vi "example_02_convert.vi"() -> ()   [LabVIEW 2015, in "lv-unit-conversion.lvlib"] (continued)
"b"=2684519.537696173, "c"=1.0, "d"=0.0, "underlying_def"="", "description"=""}, {"symbol"="hp[metric].h", "name"="metric-horsepower hour", "dimension"="L2M/T2", "is_si_unit"=TRUE, "category"="derived", "base_unit"="J", "conversion_reference"="DERIVED", "is_exact"=TRUE, "a"=0.0, "b"=2647795.5, "c"=1.0, "d"=0.0, "underlying_def"="", "description"=""}, {"symbol"="kW.h", "name"="kilowatt hour", "dimension"="L2M/T2", "is_si_unit"=TRUE, "category"="derived", "base_unit"="J", "conversion_reference"="DERIVED", "is_exact"=TRUE, "a"=0.0, "b"=3600000.0, "c"=1.0, "d"=0.0, "underlying_def"="", "description"=""}, {"symbol"="MW.h", "name"="megawatt hour", "dimension"="L2M/T2", "is_si_unit"=TRUE, "category"="derived", "base_unit"="J", "conversion_reference"="DERIVED", "is_exact"=TRUE, "a"=0.0, "b"=3600000000.0, "c"=1.0, "d"=0.0, "underlying_def"="", "description"=""}, {"symbol"="TW.h", "name"="terrawatt hour", "dimension"="L2M/T2", "is_si_unit"=TRUE, "category"="derived", "base_unit"="J", "conversion_reference"="DERIVED", "is_exact"=TRUE, "a"=0.0, "b"=3600000000000000.0, "c"=1.0, "d"=0.0, "underlying_def"="", "description"=""}, {"symbol"="1000 lbf.ft", "name"="thousand foot pound-force", "dimension"="L2M/T2", "is_si_unit"=TRUE, "category"="derived", "base_unit"="N.m", "conversion_reference"="DERIVED", "is_exact"=TRUE, "a"=0.0, "b"=1355.8179483314004, "c"=1.0, "d"=0.0, "underlying_def"="", "description"=""}, {"symbol"="daN.m", "name"="dekanewton metre", "dimension"="L2M/T2", "is_si_unit"=TRUE, "category"="derived", "base_unit"="N.m", "conversion_reference"="DERIVED", "is_exact"=TRUE, "a"=0.0, "b"=10.0, "c"=1.0, "d"=0.0, "underlying_def"="", "description"=""}, {"symbol"="dN.m", "name"="decinewton metre", "dimension"="L2M/T2", "is_si_unit"=TRUE, "category"="derived", "base_unit"="N.m", "conversion_reference"="DERIVED", "is_exact"=TRUE, "a"=0.0, "b"=0.1, "c"=1.0, "d"=0.0, "underlying_def"="", "description"=""}, {"symbol"="kgf.m", "name"="thousand gram-force metre", "dimension"="L2M/T2", "is_si_unit"=TRUE, "category"="derived", "base_unit"="N.m", "conversion_reference"="DERIVED", "is_exact"=TRUE, "a"=0.0, "b"=9.80665, "c"=1.0, "d"=0.0, "underlying_def"="", "description"=""}, {"symbol"="kN.m", "name"="kilonewton metre", "dimension"="L2M/T2", "is_si_unit"=TRUE, "category"="derived", "base_unit"="N.m", "conversion_reference"="DERIVED", "is_exact"=TRUE, "a"=0.0, "b"=1000.0, "c"=1.0, "d"=0.0, "underlying_def"="", "description"=""}, {"symbol"="lbf.ft", "name"="foot pound-force", "dimension"="L2M/T2", "is_si_unit"=TRUE, "category"="derived", "base_unit"="N.m", "conversion_reference"="DERIVED", "is_exact"=TRUE, "a"=0.0, "b"=1.3558179483314003, "c"=1.0, "d"=0.0, "underlying_def"="", "description"=""}, {"symbol"="lbf.in", "name"="inch pound-force", "dimension"="L2M/T2", "is_si_unit"=TRUE, "category"="derived", "base_unit"="N.m", "conversion_reference"="DERIVED", "is_exact"=TRUE, "a"=0.0, "b"=0.1129848290276167, "c"=1.0, "d"=0.0, "underlying_def"="", "description"=""}, {"symbol"="lbm.ft2/s2", "name"="pound-mass square foot per second squared", "dimension"="L2M/T2", "is_si_unit"=TRUE, "category"="derived", "base_unit"="N.m", "conversion_reference"="DERIVED", "is_exact"=TRUE, "a"=0.0, "b"=0.0421401100938048, "c"=1.0, "d"=0.0, "underlying_def"="", "description"=""}, {"symbol"="pdl.ft", "name"="foot poundal", "dimension"="L2M/T2", "is_si_unit"=TRUE, "category"="derived", "base_unit"="N.m", "conversion_reference"="DERIVED", "is_exact"=TRUE, "a"=0.0, "b"=0.0421401100938048, "c"=1.0, "d"=0.0, "underlying_def"="", "description"=""}, {"symbol"="tonf[US].ft", "name"="US ton-force foot", "dimension"="L2M/T2", "is_si_unit"=TRUE, "category"="derived", "base_unit"="N.m", "conversion_reference"="DERIVED", "is_exact"=TRUE, "a"=0.0, "b"=2711.635896662801, "c"=1.0, "d"=0.0, "underlying_def"="", "description"=""}, {"symbol"="tonf[US].mi", "name"="US ton-force mile", "dimension"="L2M/T2", "is_si_unit"=TRUE, "category"="derived", "base_unit"="N.m", "conversion_reference"="DERIVED", "is_exact"=TRUE, "a"=0.0, "b"=14317437.534379588, "c"=1.0, "d"=0.0, "underlying_def"="", "description"=""}, {"symbol"="aJ", "name"="attojoule", "dimension"="L2M/T2", "is_si_unit"=TRUE, "category"="prefixed", "base_unit"="J", "conversion_reference"="DERIVED", "is_exact"=TRUE, "a"=0.0, "b"=1e-18, "c"=1.0, "d"=0.0, "underlying_def"="", "description"=""}, {"symbol"="ccal[th]", "name"="hundredth of calorie", "dimension"="L2M/T2", "is_si_unit"=TRUE, "category"="prefixed", "base_unit"="J", "conversion_reference"="DERIVED", "is_exact"=TRUE, "a"=0.0, "b"=0.04184, "c"=1.0, "d"=0.0, "underlying_def"="", "description"=""}, {"symbol"="ceV", "name"="centielectronvolt", "dimension"="L2M/T2", "is_si_unit"=TRUE, "category"="prefixed", "base_unit"="J", "conversion_reference"="DERIVED", "is_exact"=TRUE, "a"=0.0, "b"=1.602176487e-21, "c"=1.0, "d"=0.0, "underlying_def"="", "description"=""}, {"symbol"="cJ", "name"="centijoule", "dimension"="L2M/T2", "is_si_unit"=TRUE, "category"="prefixed", "base_unit"="J", "conversion_reference"="DERIVED", "is_exact"=TRUE, "a"=0.0, "b"=0.01, "c"=1.0, "d"=0.0, "underlying_def"="", "description"=""}, {"symbol"="dcal[th]", "name"="tenth of calorie", "dimension"="L2M/T2", "is_si_unit"=TRUE, "category"="prefixed", "base_unit"="J", "conversion_reference"="DERIVED", "is_exact"=TRUE, "a"=0.0, "b"=0.4184, "c"=1.0, "d"=0.0, "underlying_def"="", "description"=""}, {"symbol"="deV", "name"="decielectronvolt", "dimension"="L2M/T2", "is_si_unit"=TRUE, "category"="prefixed", "base_unit"="J", "conversion_reference"="DERIVED", "is_exact"=TRUE, "a"=0.0, "b"=1.602176487e-20, "c"=1.0, "d"=0.0, "underlying_def"="", "description"=""}, {"symbol"="dJ", "name"="decijoule", "dimension"="L2M/T2", "is_si_unit"=TRUE, "category"="prefixed", "base_unit"="J", "conversion_reference"="DERIVED", "is_exact"=TRUE, "a"=0.0, "b"=0.1, "c"=1.0, "d"=0.0, "underlying_def"="", "description"=""}, {"symbol"="Ecal[th]", "name"="million million million calorie", "dimension"="L2M/T2", "is_si_unit"=TRUE, "category"="prefixed", "base_unit"="J", "conversion_reference"="DERIVED", "is_exact"=TRUE, "a"=0.0, "b"=4.184e+18, "c"=1.0, "d"=0.0, "underlying_def"="", "description"=""}, {"symbol"="EeV", "name"="exaelectronvolt", "dimension"="L2M/T2", "is_si_unit"=TRUE, "category"="prefixed", "base_unit"="J", "conversion_reference"="DERIVED", "is_exact"=TRUE, "a"=0.0, "b"=0.1602176487, "c"=1.0, "d"=0.0, "underlying_def"="", "description"=""}, {"symbol"="EJ", "name"="exajoule", "dimension"="L2M/T2", "is_si_unit"=TRUE, "category"="prefixed", "base_unit"="J", "conversion_reference"="DERIVED", "is_exact"=TRUE, "a"=0.0, "b"=1e+18, "c"=1.0, "d"=0.0, "underlying_def"="", "description"=""}, {"symbol"="fcal[th]", "name"="femtocalorie", "dimension"="L2M/T2", "is_si_unit"=TRUE, "category"="prefixed", "base_unit"="J", "conversion_reference"="DERIVED", "is_exact"=TRUE, "a"=0.0, "b"=4.184e-15, "c"=1.0, "d"=0.0, "underlying_def"="", "description"=""}, {"symbol"="feV", "name"="femtoelectronvolt", "dimension"="L2M/T2", "is_si_unit"=TRUE, "category"="prefixed", "base_unit"="J", "conversion_reference"="DERIVED", "is_exact"=TRUE, "a"=0.0, "b"=1.602176487e-34, "c"=1.0, "d"=0.0, "underlying_def"="", "description"=""}, {"symbol"="fJ", "name"="femtojoule", "dimension"="L2M/T2", "is_si_unit"=TRUE, "category"="prefixed", "base_unit"="J", "conversion_reference"="DERIVED", "is_exact"=TRUE, "a"=0.0, "b"=1e-15, "c"=1.0, "d"=0.0, "underlying_def"="", "description"=""}, {"symbol"="Gcal[th]", "name"="thousand million calorie", "dimension"="L2M/T2", "is_si_unit"=TRUE, "category"="prefixed", "base_unit"="J", "conversion_reference"="DERIVED", "is_exact"=TRUE, "a"=0.0, "b"=4184000000.0, "c"=1.0, "d"=0.0, "underlying_def"="", "description"=""}, {"symbol"="GeV", "name"="gigaelectronvolt", "dimension"="L2M/T2", "is_si_unit"=TRUE, "category"="prefixed", "base_unit"="J", "conversion_reference"="DERIVED", "is_exact"=TRUE, "a"=0.0, "b"=1.602176487e-10, "c"=1.0, "d"=0.0, "underlying_def"="", "description"=""}, {"symbol"="GJ", "name"="gigajoule", "dimension"="L2M/T2", "is_si_unit"=TRUE, "category"="prefixed", "base_unit"="J", "conversion_reference"="DERIVED", "is_exact"=TRUE, "a"=0.0, "b"=1000000000.0, "c"=1.0, "d"=0.0, "underlying_def"="", "description"=""}, {"symbol"="kcal[th]", "name"="thousand calorie", "dimension"="L2M/T2", "is_si_unit"=TRUE, "category"="prefixed", "base_unit"="J", "conversion_reference"="DERIVED", "is_exact"=TRUE, "a"=0.0, "b"=4184.0, "c"=1.0, "d"=0.0, "underlying_def"="", "description"="thermochemical calorie"}, {"symbol"="keV", "name"="kiloelectronvolt", "dimension"="L2M/T2", "is_si_unit"=TRUE, "category"="prefixed", "base_unit"="J", "conversion_reference"="DERIVED", "is_exact"=TRUE, "a"=0.0, "b"=1.602176487e-16, "c"=1.0, "d"=0.0, "underlying_def"="", "description"=""}, {"symbol"="kJ", "name"="kilojoule", "dimension"="L2M/T2", "is_si_unit"=TRUE, "category"="prefixed", "base_unit"="J", "conversion_reference"="DERIVED", "is_exact"=TRUE, "a"=0.0, "b"=1000.0, "c"=1.0, "d"=0.0, "underlying_def"="", "description"=""}, {"symbol"="mcal[th]", "name"="thousandth of calorie", "dimension"="L2M/T2", "is_si_unit"=TRUE, "category"="prefixed", "base_unit"="J", "conversion_reference"="DERIVED", "is_exact"=TRUE, "a"=0.0, "b"=0.004184, "c"=1.0, "d"=0.0, "underlying_def"="", "description"=""}, {"symbol"="Mcal[th]", "name"="million calorie", "dimension"="L2M/T2", "is_si_unit"=TRUE, "category"="prefixed", "base_unit"="J", "conversion_reference"="DERIVED", "is_exact"=TRUE, "a"=0.0, "b"=4184000.0, "c"=1.0, "d"=0.0, "underlying_def"="", "description"=""}, {"symbol"="MeV", "name"="megaelectronvolt", "dimension"="L2M/T2", "is_si_unit"=TRUE, "category"="prefixed", "base_unit"="J", "conversion_reference"="DERIVED", "is_exact"=TRUE, "a"=0.0, "b"=1.602176487e-13, "c"=1.0, "d"=0.0, "underlying_def"="", "description"=""}, {"symbol"="meV", "name"="millielectronvolt", "dimension"="L2M/T2", "is_si_unit"=TRUE, "category"="prefixed", "base_unit"="J", "conversion_reference"="DERIVED", "is_exact"=TRUE, "a"=0.0, "b"=1.602176487e-22, "c"=1.0, "d"=0.0, "underlying_def"="", "description"=""}, {"symbol"="mJ", "name"="millijoule", "dimension"="L2M/T2", "is_si_unit"=TRUE, "category"="prefixed", "base_unit"="J", "conversion_reference"="DERIVED", "is_exact"=TRUE, "a"=0.0, "b"=0.001, "c"=1.0, "d"=0.0, "underlying_def"="", "description"=""}, {"symbol"="MJ", "name"="megajoule", "dimension"="L2M/T2", "is_si_unit"=TRUE, "category"="prefixed", "base_unit"="J", "conversion_reference"="DERIVED", "is_exact"=TRUE, "a"=0.0, "b"=1000000.0, "c"=1.0, "d"=0.0, "underlying_def"="", "description"=""}, {"symbol"="ncal[th]", "name"="nanocalorie", "dimension"="L2M/T2", "is_si_unit"=TRUE, "category"="prefixed", "base_unit"="J", "conversion_reference"="DERIVED", "is_exact"=TRUE, "a"=0.0, "b"=4.184e-09, "c"=1.0, "d"=0.0, "underlying_def"="", "description"=""}, {"symbol"="neV", "name"="nanoelectronvolt", "dimension"="L2M/T2", "is_si_unit"=TRUE, "category"="prefixed", "base_unit"="J", "conversion_reference"="DERIVED", "is_exact"=TRUE, "a"=0.0, "b"=1.602176487e-28, "c"=1.0, "d"=0.0, "underlying_def"="", "description"=""}, {"symbol"="nJ", "name"="nanojoule", "dimension"="L2M/T2", "is_si_unit"=TRUE, "category"="prefixed", "base_unit"="J", "conversion_reference"="DERIVED", "is_exact"=TRUE, "a"=0.0, "b"=1e-09, "c"=1.0, "d"=0.0, "underlying_def"="", "description"=""}, {"symbol"="pcal[th]", "name"="picocalorie", "dimension"="L2M/T2", "is_si_unit"=TRUE, "category"="prefixed", "base_unit"="J", "conversion_reference"="DERIVED", "is_exact"=TRUE, "a"=0.0, "b"=4.184e-12, "c"=1.0, "d"=0.0, "underlying_def"="", "description"=""}, {"symbol"="peV", "name"="picoelectronvolt", "dimension"="L2M/T2", "is_si_unit"=TRUE, "category"="prefixed", "base_unit"="J", "conversion_reference"="DERIVED", "is_exact"=TRUE, "a"=0.0, "b"=1.602176487e-31, "c"=1.0, "d"=0.0, "underlying_def"="", "description"=""}, {"symbol"="pJ", "name"="picojoule", "dimension"="L2M/T2", "is_si_unit"=TRUE, "category"="prefixed", "base_unit"="J", "conversion_reference"="DERIVED", "is_exact"=TRUE, "a"=0.0, "b"=1e-12, "c"=1.0, "d"=0.0, "underlying_def"="", "description"=""}, {"symbol"="Tcal[th]", "name"="million million calorie", "dimension"="L2M/T2", "is_si_unit"=TRUE, "category"="prefixed", "base_unit"="J", "conversion_reference"="DERIVED", "is_exact"=TRUE, "a"=0.0, "b"=4184000000000.0, "c"=1.0, "d"=0.0, "underlying_def"="", "description"=""}, {"symbol"="TeV", "name"="teraelectronvolt", "dimension"="L2M/T2", "is_si_unit"=TRUE, "category"="prefixed", "base_unit"="J", "conversion_reference"="DERIVED", "is_exact"=TRUE, "a"=0.0, "b"=1.602176487e-07, "c"=1.0, "d"=0.0, "underlying_def"="", "description"=""}, {"symbol"="TJ", "name"="terajoule", "dimension"="L2M/T2", "is_si_unit"=TRUE, "category"="prefixed", "base_unit"="J", "conversion_reference"="DERIVED", "is_exact"=TRUE, "a"=0.0, "b"=1000000000000.0, "c"=1.0, "d"=0.0, "underlying_def"="", "description"=""}, {"symbol"="ucal[th]", "name"="millionth of calorie", "dimension"="L2M/T2", "is_si_unit"=TRUE, "category"="prefixed", "base_unit"="J", "conversion_reference"="DERIVED", "is_exact"=TRUE, "a"=0.0, "b"=4.184e-06, "c"=1.0, "d"=0.0, "underlying_def"="", "description"=""}, {"symbol"="ueV", "name"="microelectronvolt", "dimension"="L2M/T2", "is_si_unit"=TRUE, "category"="prefixed", "base_unit"="J", "conversion_reference"="DERIVED", "is_exact"=TRUE, "a"=0.0, "b"=1.602176487e-25, "c"=1.0, "d"=0.0, "underlying_def"="", "description"=""}, {"symbol"="uJ", "name"="microjoule", "dimension"="L2M/T2", "is_si_unit"=TRUE, "category"="prefixed", "base_unit"="J", "conversion_reference"="DERIVED", "is_exact"=TRUE, "a"=0.0, "b"=1e-06, "c"=1.0, "d"=0.0, "underlying_def"="", "description"=""}, {"symbol"="W", "name"="watt", "dimension"="L2M/T3", "is_si_unit"=TRUE, "category"="atom-special", "base_unit"="", "conversion_reference"="", "is_exact"=FALSE, "a"=0.0, "b"=0.0, "c"=0.0, "d"=0.0, "underlying_def"="J/s", "description"="The power that represents a rate of energy transfer of 1 J/s."}, {"symbol"="hp", "name"="horsepower", "dimension"="L2M/T3", "is_si_unit"=TRUE, "category"="atom", "base_unit"="W", "conversion_reference"="UK-1995", "is_exact"=TRUE, "a"=0.0, "b"=745.6998715822702, "c"=1.0, "d"=0.0, "underlying_def"="550 lbf.ft/s", "description"="The mechanical horsepower, also known as imperial horsepower, of exactly 550 foot pound-force per second.\n\t\t\t"}, {"symbol"="hp[elec]", "name"="electric-horsepower", "dimension"="L2M/T3", "is_si_unit"=TRUE, "category"="atom", "base_unit"="W", "conversion_reference"="NIST-SI", "is_exact"=TRUE, "a"=0.0, "b"=746.0, "c"=1.0, "d"=0.0, "underlying_def"="746 W", "description"="The horsepower used for electrical machines is defined as exactly 746 W. \n\t\t\t\tOutside the United States watts are generally used for electrical power applications.\n\t\t\t"}, {"symbol"="hp[hyd]", "name"="hydraulic-horsepower", "dimension"="L2M/T3", "is_si_unit"=TRUE, "category"="atom", "base_unit"="W", "conversion_reference"="NIST-SI", "is_exact"=TRUE, "a"=0.0, "b"=746.043, "c"=1.0, "d"=0.0, "underlying_def"="", "description"="Also called water horsepower (from NIST-SI). \n\t\t\t\tCommonly calculated with the equation HHP=P*Q/1714, where P stands for pressure in pounds per square \n\t\t\t\tinch, Q stands for flow rate in gallons per minute, and 1714 is a conversion factor necessary to \n\t\t\t\tyield HHP in terms of horsepower (from Schlumberger Oilfield Glossary).\n\t\t\t"}, {"symbol"="hp[metric]", "name"="metric-horsepower", "dimension"="L2M/T3", "is_si_unit"=TRUE, "category"="atom", "base_unit"="W", "conversion_reference"="EEC-71-354", "is_exact"=TRUE, "a"=0.0, "b"=735.49875, "c"=1.0, "d"=0.0, "underlying_def"="", "description"="The power to raise a mass of 75 kilograms against the earth's gravitational force over a distance of \n\t\t\t\tone metre in one second. \n\t\t\t\tAlso known as the Pferdestarke (PS), the paardenkracht (pk), the cheval vapeur (CV) and the cavallo \n\t\t\t\tvapore (cv).\n\t\t\t"}, {"symbol"="tonRefrig", "name"="ton-refrigeration", "dimension"="L2M/T3", "is_si_unit"=TRUE, "category"="atom", "base_unit"="W", "conversion_reference"="NIST-SI", "is_exact"=TRUE, "a"=0.0, "b"=12660670.23144, "c"=3600.0, "d"=0.0, "underlying_def"="12000 Btu[IT]/h", "description"="A ton of refrigeration is 12,000 (international table) Btu/h."}, {"symbol"="J/s", "name"="joule per second", "dimension"="L2M/T3", "is_si_unit"=TRUE, "category"="derived", "base_unit"="", "conversion_reference"="", "is_exact"=FALSE, "a"=0.0, "b"=0.0, "c"=0.0, "d"=0.0, "underlying_def"="W", "description"=""}, {"symbol"="1E6 Btu[IT]/h", "name"="million BTU per hour", "dimension"="L2M/T3", "is_si_unit"=TRUE, "category"="derived", "base_unit"="J/s", "conversion_reference"="DERIVED", "is_exact"=TRUE, "a"=0.0, "b"=1055055852.62, "c"=3600.0, "d"=0.0, "underlying_def"="", "description"=""}, {"symbol"="Btu[IT]/h", "name"="BTU per hour", "dimension"="L2M/T3", "is_si_unit"=TRUE, "category"="derived", "base_unit"="J/s", "conversion_reference"="DERIVED", "is_exact"=TRUE, "a"=0.0, "b"=1055.05585262, "c"=3600.0, "d"=0.0, "underlying_def"="", "description"=""}, {"symbol"="Btu[IT]/min", "name"="BTU per minute", "dimension"="L2M/T3", "is_si_unit"=TRUE, "category"="derived", "base_unit"="J/s", "conversion_reference"="DERIVED", "is_exact"=TRUE, "a"=0.0, "b"=1055.05585262, "c"=60.0, "d"=0.0, "underlying_def"="", "description"=""}, {"symbol"="Btu[IT]/s", "name"="BTU per second", "dimension"="L2M/T3", "is_si_unit"=TRUE, "category"="derived", "base_unit"="J/s", "conversion_reference"="DERIVED", "is_exact"=TRUE, "a"=0.0, "b"=1055.05585262, "c"=1.0, "d"=0.0, "underlying_def"="", "description"=""}, {"symbol"="cal[th]/h", "name"="calorie per hour", "dimension"="L2M/T3", "is_si_unit"=TRUE, "category"="derived", "base_unit"="J/s", "conversion_reference"="DERIVED", "is_exact"=TRUE, "a"=0.0, "b"=4.184, "c"=3600.0, "d"=0.0, "underlying_def"="", "description"=""}, {"symbol"="EJ/a", "name"="exajoule per julian-year", "dimension"="L2M/T3", "is_si_unit"=TRUE, "category"="derived", "base_unit"="J/s", "conversion_reference"="DERIVED", "is_exact"=TRUE, "a"=0.0, "b"=1e+18, "c"=31557600.0, "d"=0.0, "underlying_def"="", "description"=""}, {"symbol"="erg/a", "name"="erg per julian-year", "dimension"="L2M/T3", "is_si_unit"=TRUE, "category"="derived", "base_unit"="J/s", "conversion_reference"="DERIVED", "is_exact"=TRUE, "a"=0.0, "b"=1e-07, "c"=31557600.0, "d"=0.0, "underlying_def"="", "description"=""}, {"symbol"="kcal[th]/h", "name"="thousand calorie per hour", "dimension"="L2M/T3", "is_si_unit"=TRUE, "category"="derived", "base_unit"="J/s", "conversion_reference"="DERIVED", "is_exact"=TRUE, "a"=0.0, "b"=4184.0, "c"=3600.0, "d"=0.0, "underlying_def"="", "description"=""}, {"symbol"="lbf.ft/min", "name"="foot pound-force per minute", "dimension"="L2M/T3", "is_si_unit"=TRUE, "category"="derived", "base_unit"="J/s", "conversion_reference"="DERIVED", "is_exact"=TRUE, "a"=0.0, "b"=1.3558179483314003, "c"=60.0, "d"=0.0, "underlying_def"="", "description"=""}, {"symbol"="lbf.ft/s", "name"="foot pound-force per second", "dimension"="L2M/T3", "is_si_unit"=TRUE, "category"="derived", "base_unit"="J/s", "conversion_reference"="DERIVED", "is_exact"=TRUE, "a"=0.0, "b"=1.3558179483314003, "c"=1.0, "d"=0.0, "underlying_def"="", "description"=""}, {"symbol"="MJ/a", "name"="megajoule per julian-year", "dimension"="L2M/T3", "is_si_unit"=TRUE, "category"="derived", "base_unit"="J/s", "conversion_reference"="DERIVED", "is_exact"=TRUE, "a"=0.0, "b"=1000000.0, "c"=31557600.0, "d"=0.0, "underlying_def"="", "description"=""}, {"symbol"="quad/a", "name"="quad per julian-year", "dimension"="L2M/T3", "is_si_unit"=TRUE, "category"="derived", "base_unit"="J/s", "conversion_reference"="DERIVED", "is_exact"=TRUE, "a"=0.0, "b"=1.05505585262e+18, "c"=31557600.0, "d"=0.0, "underlying_def"="", "description"=""}, {"symbol"="TJ/a", "name"="terajoule per julian-year", "dimension"="L2M/T3", "is_si_unit"=TRUE, "category"="derived", "base_unit"="J/s", "conversion_reference"="DERIVED", "is_exact"=TRUE, "a"=0.0, "b"=1000000000000.0, "c"=31557600.0, "d"=0.0, "underlying_def"="", "description"=""}, {"symbol"="ucal[th]/s", "name"="millionth of calorie per second", "dimension"="L2M/T3", "is_si_unit"=TRUE, "category"="derived", "base_unit"="J/s", "conversion_reference"="DERIVED", "is_exact"=TRUE, "a"=0.0, "b"=4.184e-06, "c"=1.0, "d"=0.0, "underlying_def"="", "description"=""}, {"symbol"="cW", "name"="centiwatt", "dimension"="L2M/T3", "is_si_unit"=TRUE, "category"="prefixed", "base_unit"="W", "conversion_reference"="DERIVED", "is_exact"=TRUE, "a"=0.0, "b"=0.01, "c"=1.0, "d"=0.0, "underlying_def"="", "description"=""}, {"symbol"="dW", "name"="deciwatt", "dimension"="L2M/T3", "is_si_unit"=TRUE, "category"="prefixed", "base_unit"="W", "conversion_reference"="DERIVED", "is_exact"=TRUE, "a"=0.0, "b"=0.1, "c"=1.0, "d"=0.0, "underlying_def"="", "description"=""}, {"symbol"="EW", "name"="exawatt", "dimension"="L2M/T3", "is_si_unit"=TRUE, "category"="prefixed", "base_unit"="W", "conversion_reference"="DERIVED", "is_exact"=TRUE, "a"=0.0, "b"=1e+18, "c"=1.0, "d"=0.0, "underlying_def"="", "description"=""}, {"symbol"="fW", "name"="femtowatt", "dimension"="L2M/T3", "is_si_unit"=TRUE, "category"="prefixed", "base_unit"="W", "conversion_reference"="DERIVED", "is_exact"=TRUE, "a"=0.0, "b"=1e-15, "c"=1.0, "d"=0.0, "underlying_def"="", "description"=""}, {"symbol"="GW", "name"="gigawatt", "dimension"="L2M/T3", "is_si_unit"=TRUE, "category"="prefixed", "base_unit"="W", "conversion_reference"="DERIVED", "is_exact"=TRUE, "a"=0.0, "b"=1000000000.0, "c"=1.0, "d"=0.0, "underlying_def"="", "description"=""}, {"symbol"="kW", "name"="kilowatt", "dimension"="L2M/T3", "is_si_unit"=TRUE, "category"="prefixed", "base_unit"="W", "conversion_reference"="DERIVED", "is_exact"=TRUE, "a"=0.0, "b"=1000.0, "c"=1.0, "d"=0.0, "underlying_def"="", "description"=""}, {"symbol"="mW", "name"="milliwatt", "dimension"="L2M/T3", "is_si_unit"=TRUE, "category"="prefixed", "base_unit"="W", "conversion_reference"="DERIVED", "is_exact"=TRUE, "a"=0.0, "b"=0.001, "c"=1.0, "d"=0.0, "underlying_def"="", "description"=""}, {"symbol"="MW", "name"="megawatt", "dimension"="L2M/T3", "is_si_unit"=TRUE, "category"="prefixed", "base_unit"="W", "conversion_reference"="DERIVED", "is_exact"=TRUE, "a"=0.0, "b"=1000000.0, "c"=1.0, "d"=0.0, "underlying_def"="", "description"=""}, {"symbol"="nW", "name"="nanowatt", "dimension"="L2M/T3", "is_si_unit"=TRUE, "category"="prefixed", "base_unit"="W", "conversion_reference"="DERIVED", "is_exact"=TRUE, "a"=0.0, "b"=1e-09, "c"=1.0, "d"=0.0, "underlying_def"="", "description"=""}, {"symbol"="pW", "name"="picowatt", "dimension"="L2M/T3", "is_si_unit"=TRUE, "category"="prefixed", "base_unit"="W", "conversion_reference"="DERIVED", "is_exact"=TRUE, "a"=0.0, "b"=1e-12, "c"=1.0, "d"=0.0, "underlying_def"="", "description"=""}, {"symbol"="TW", "name"="terawatt", "dimension"="L2M/T3", "is_si_unit"=TRUE, "category"="prefixed", "base_unit"="W", "conversion_reference"="DERIVED", "is_exact"=TRUE, "a"=0.0, "b"=1000000000000.0, "c"=1.0, "d"=0.0, "underlying_def"="", "description"=""}, {"symbol"="uW", "name"="microwatt", "dimension"="L2M/T3", "is_si_unit"=TRUE, "category"="prefixed", "base_unit"="W", "conversion_reference"="DERIVED", "is_exact"=TRUE, "a"=0.0, "b"=1e-06, "c"=1.0, "d"=0.0, "underlying_def"="", "description"=""}, {"symbol"="m/Pa", "name"="metre per Pascal", "dimension"="L2T2/M", "is_si_unit"=TRUE, "category"="derived", "base_unit"="", "conversion_reference"="", "is_exact"=FALSE, "a"=0.0, "b"=0.0, "c"=0.0, "d"=0.0, "underlying_def"="", "description"=""}, {"symbol"="ft/psi", "name"="foot per psi", "dimension"="L2T2/M", "is_si_unit"=TRUE, "category"="derived", "base_unit"="m/Pa", "conversion_reference"="DERIVED", "is_exact"=TRUE, "a"=0.0, "b"=0.000196644768, "c"=4.4482216152605, "d"=0.0, "underlying_def"="", "description"=""}, {"symbol"="m/kPa", "name"="metre per kilopascal", "dimension"="L2T2/M", "is_si_unit"=TRUE, "category"="derived", "base_unit"="m/Pa", "conversion_reference"="DERIVED", "is_exact"=TRUE, "a"=0.0, "b"=0.001, "c"=1.0, "d"=0.0, "underlying_def"="", "description"=""}, {"symbol"="bbl", "name"="barrel", "dimension"="L3", "is_si_unit"=TRUE, "category"="atom", "base_unit"="m3", "conversion_reference"="NIST-SI", "is_exact"=TRUE, "a"=0.0, "b"=0.158987294928, "c"=1.0, "d"=0.0, "underlying_def"="42 gal[US]", "description"="42 US gallons. \n\t\t\t\t1 barrel of oil (bbl) is defined as exactly 42 US liquid gallons. \n\t\t\t\t1 US liquid gallon is defined as exactly 231 cubic inches (see NIST-130 reference). \n\t\t\t\t1 inch is defined as exactly 0.0254 metres. \n\t\t\t\tTherefore, 1 bbl = (42 x 231 x 0.0254**3) m3 = 0.158987294928 m3 exactly. \n\t\t\t\tNote that this definition is based in the international inch and NOT the older US survey inch.\n\t\t\t"}, {"symbol"="floz[UK]", "name"="UK fluid-ounce", "dimension"="L3", "is_si_unit"=TRUE, "category"="atom", "base_unit"="m3", "conversion_reference"="UK-1985", "is_exact"=TRUE, "a"=0.0, "b"=0.00454609, "c"=160.0, "d"=0.0, "underlying_def"="1/20 pt[UK]", "description"="United Kingdom 1/20 of UK pint. \n\t\t\t\tTherefore, 1/160 of UK gallon or (1/160)* 4.54609 cubic decimetres. \n\t\t\t\tFrom UK-1985.\n\t\t\t"}, {"symbol"="floz[US]", "name"="US fluid-ounce", "dimension"="L3", "is_si_unit"=TRUE, "category"="atom", "base_unit"="m3", "conversion_reference"="NIST-44", "is_exact"=TRUE, "a"=0.0, "b"=0.003785411784, "c"=128.0, "d"=0.0, "underlying_def"="1/128 gal[US]", "description"="1/16 of US pint which is 1/8 of US gallon. Therefore, 1/128 of US gallon."}, {"symbol"="gal[UK]", "name"="UK gallon", "dimension"="L3", "is_si_unit"=TRUE, "category"="atom", "base_unit"="m3", "conversion_reference"="UK-1985", "is_exact"=TRUE, "a"=0.0, "b"=0.00454609, "c"=1.0, "d"=0.0, "underlying_def"="4.54609 dm3", "description"="United Kingdom Imperial gallon. \n\t\t\t\tIn Great Britain, a unit of capacity, by the Weights and Measures Act of 1985, exactly \"4.54609 \n\t\t\t\tcubic decimeters\".\n\t\t\t"}, {"symbol"="gal[US]", "name"="US gallon", "dimension"="L3", "is_si_unit"=TRUE, "category"="atom", "base_unit"="m3", "conversion_reference"="NIST-44", "is_exact"=TRUE, "a"=0.0, "b"=0.003785411784, "c"=1.0, "d"=0.0, "underlying_def"="231 in3", "description"="The United States liquid gallon is legally defined as 231 cubic inches, and is equal to exactly \n\t\t\t\t3.785411784 litres. \n\t\t\t\tAuthorized tables, US Code, Title 15, chapter 6, subchapter I, section 205.\n\t\t\t"}, {"symbol"="L", "name"="litre", "dimension"="L3", "is_si_unit"=TRUE, "category"="atom-allowed", "base_unit"="m3", "conversion_reference"="NIST-44", "is_exact"=TRUE, "a"=0.0, "b"=0.001, "c"=1.0, "d"=0.0, "underlying_def"="dm3", "description"="Liquid volume. \n\t\t\t\tIn the US, this is called a liter. \n\t\t\t\tBy action of the 12th General Conference on Weights and Measures (1964), the liter is a special name \n\t\t\t\tfor the cubic decimeter.\n\t\t\t"}, {"symbol"="pt[UK]", "name"="UK pint", "dimension"="L3", "is_si_unit"=TRUE, "category"="atom", "base_unit"="m3", "conversion_reference"="UK-1985", "is_exact"=TRUE, "a"=0.0, "b"=0.00454609, "c"=8.0, "d"=0.0, "underlying_def"="1/8 gal[UK]", "description"="There are two pints to one quart"}, {"symbol"="pt[US]", "name"="US pint", "dimension"="L3", "is_si_unit"=TRUE, "category"="atom", "base_unit"="m3", "conversion_reference"="NIST-44", "is_exact"=TRUE, "a"=0.0, "b"=0.003785411784, "c"=8.0, "d"=0.0, "underlying_def"="1/8 gal[US]", "description"="There are two pints to one quart"}, {"symbol"="qt[UK]", "name"="UK quart", "dimension"="L3", "is_si_unit"=TRUE, "category"="atom", "base_unit"="m3", "conversion_reference"="UK-1985", "is_exact"=TRUE, "a"=0.0, "b"=0.00454609, "c"=4.0, "d"=0.0, "underlying_def"="1/4 gal[UK]", "description"="There are four quarts to one gallon."}, {"symbol"="qt[US]", "name"="US quart", "dimension"="L3", "is_si_unit"=TRUE, "category"="atom", "base_unit"="m3", "conversion_reference"="NIST-44", "is_exact"=TRUE, "a"=0.0, "b"=0.003785411784, "c"=4.0, "d"=0.0, "underlying_def"="1/4 gal[US]", "description"="There are four quarts to one gallon."}, {"symbol"="TD[API].m", "name"="teradarcy-API metre", "dimension"="L3", "is_si_unit"=TRUE, "category"="derived", "base_unit"="", "conversion_reference"="", "is_exact"=FALSE, "a"=0.0, "b"=0.0, "c"=0.0, "d"=0.0, "underlying_def"="m3", "description"=""}, {"symbol"="1000 bbl", "name"="thousand barrel", "dimension"="L3", "is_si_unit"=TRUE, "category"="derived", "base_unit"="m3", "conversion_reference"="DERIVED", "is_exact"=TRUE, "a"=0.0, "b"=158.987294928, "c"=1.0, "d"=0.0, "underlying_def"="", "description"=""}, {"symbol"="1000 ft3", "name"="thousand cubic foot", "dimension"="L3", "is_si_unit"=TRUE, "category"="derived", "base_unit"="m3", "conversion_reference"="DERIVED", "is_exact"=TRUE, "a"=0.0, "b"=28.316846592, "c"=1.0, "d"=0.0, "underlying_def"="", "description"=""}, {"symbol"="1000 gal[UK]", "name"="thousand UK gallon", "dimension"="L3", "is_si_unit"=TRUE, "category"="derived", "base_unit"="m3", "conversion_reference"="DERIVED", "is_exact"=TRUE, "a"=0.0, "b"=4.54609, "c"=1.0, "d"=0.0, "underlying_def"="", "description"=""}, {"symbol"="1000 gal[US]", "name"="thousand US gallon", "dimension"="L3", "is_si_unit"=TRUE, "category"="derived", "base_unit"="m3", "conversion_reference"="DERIVED", "is_exact"=TRUE, "a"=0.0, "b"=3.785411784, "c"=1.0, "d"=0.0, "underlying_def"="", "description"=""}, {"symbol"="1000 m3", "name"="thousand cubic metre", "dimension"="L3", "is_si_unit"=TRUE, "category"="derived", "base_unit"="m3", "conversion_reference"="DERIVED", "is_exact"=TRUE, "a"=0.0, "b"=1000.0, "c"=1.0, "d"=0.0, "underlying_def"="", "description"=""}, {"symbol"="1E12 ft3", "name"="million million cubic foot", "dimension"="L3", "is_si_unit"=TRUE, "category"="derived", "base_unit"="m3", "conversion_reference"="DERIVED", "is_exact"=TRUE, "a"=0.0, "b"=28316846592.0, "c"=1.0, "d"=0.0, "underlying_def"="", "description"=""}, {"symbol"="1E6 bbl", "name"="million barrel", "dimension"="L3", "is_si_unit"=TRUE, "category"="derived", "base_unit"="m3", "conversion_reference"="DERIVED", "is_exact"=TRUE, "a"=0.0, "b"=158987.294928, "c"=1.0, "d"=0.0, "underlying_def"="", "description"=""}, {"symbol"="1E6 ft3", "name"="million cubic foot", "dimension"="L3", "is_si_unit"=TRUE, "category"="derived", "base_unit"="m3", "conversion_reference"="DERIVED", "is_exact"=TRUE, "a"=0.0, "b"=28316.846592, "c"=1.0, "d"=0.0, "underlying_def"="", "description"=""}, {"symbol"="1E-6 gal[US]", "name"="millionth of US gallon", "dimension"="L3", "is_si_unit"=TRUE, "category"="derived", "base_unit"="m3", "conversion_reference"="DERIVED", "is_exact"=TRUE, "a"=0.0, "b"=3.785411784e-09, "c"=1.0, "d"=0.0, "underlying_def"="", "description"=""}, {"symbol"="1E6 m3", "name"="million cubic metre", "dimension"="L3", "is_si_unit"=TRUE, "category"="derived", "base_unit"="m3", "conversion_reference"="DERIVED", "is_exact"=TRUE, "a"=0.0, "b"=1000000.0, "c"=1.0, "d"=0.0, "underlying_def"="", "description"=""}, {"symbol"="1E9 bbl", "name"="thousand million barrel", "dimension"="L3", "is_si_unit"=TRUE, "category"="derived", "base_unit"="m3", "conversion_reference"="DERIVED", "is_exact"=TRUE, "a"=0.0, "b"=158987294.928, "c"=1.0, "d"=0.0, "underlying_def"="", "description"=""}, {"symbol"="1E9 ft3", "name"="thousand million cubic foot", "dimension"="L3", "is_si_unit"=TRUE, "category"="derived", "base_unit"="m3", "conversion_reference"="DERIVED", "is_exact"=TRUE, "a"=0.0, "b"=28316846.592, "c"=1.0, "d"=0.0, "underlying_def"="", "description"=""}, {"symbol"="acre.ft", "name"="acre foot", "dimension"="L3", "is_si_unit"=TRUE, "category"="derived", "base_unit"="m3", "conversion_reference"="DERIVED", "is_exact"=TRUE, "a"=0.0, "b"=19119006720.0, "c"=15499969.0, "d"=0.0, "underlying_def"="", "description"=""}, {"symbol"="cm3", "name"="cubic centimetre", "dimension"="L3", "is_si_unit"=TRUE, "category"="derived", "base_unit"="m3", "conversion_reference"="DERIVED", "is_exact"=TRUE, "a"=0.0, "b"=1e-06, "c"=1.0, "d"=0.0, "underlying_def"="", "description"=""}, {"symbol"="dm3", "name"="cubic decimetre", "dimension"="L3", "is_si_unit"=TRUE, "category"="derived", "base_unit"="m3", "conversion_reference"="DERIVED", "is_exact"=TRUE, "a"=0.0, "b"=0.001, "c"=1.0, "d"=0.0, "underlying_def"="", "description"=""}, {"symbol"="ha.m", "name"="hectare metre", "dimension"="L3", "is_si_unit"=TRUE, "category"="derived", "base_unit"="m3", "conversion_reference"="DERIVED", "is_exact"=TRUE, "a"=0.0, "b"=10000.0, "c"=1.0, "d"=0.0, "underlying_def"="", "description"=""}, {"symbol"="km3", "name"="cubic kilometre", "dimension"="L3", "is_si_unit"=TRUE, "category"="derived", "base_unit"="m3", "conversion_reference"="DERIVED", "is_exact"=TRUE, "a"=0.0, "b"=1000000000.0, "c"=1.0, "d"=0.0, "underlying_def"="", "description"=""}, {"symbol"="mm3", "name"="cubic millimetre", "dimension"="L3", "is_si_unit"=TRUE, "category"="derived", "base_unit"="m3", "conversion_reference"="DERIVED", "is_exact"=TRUE, "a"=0.0, "b"=1e-09, "c"=1.0, "d"=0.0, "underlying_def"="", "description"=""}, {"symbol"="um2.m", "name"="square micrometre metre", "dimension"="L3", "is_si_unit"=TRUE, "category"="derived", "base_unit"="m3", "conversion_reference"="DERIVED", "is_exact"=TRUE, "a"=0.0, "b"=1e-12, "c"=1.0, "d"=0.0, "underlying_def"="", "description"=""}, {"symbol"="D.ft", "name"="darcy foot", "dimension"="L3", "is_si_unit"=TRUE, "category"="derived", "base_unit"="TD[API].m", "conversion_reference"="DERIVED", "is_exact"=TRUE, "a"=0.0, "b"=3.048e-13, "c"=1.01325, "d"=0.0, "underlying_def"="", "description"=""}, {"symbol"="D.m", "name"="darcy metre", "dimension"="L3", "is_si_unit"=TRUE, "category"="derived", "base_unit"="TD[API].m", "conversion_reference"="DERIVED", "is_exact"=TRUE, "a"=0.0, "b"=1e-12, "c"=1.01325, "d"=0.0, "underlying_def"="", "description"=""}, {"symbol"="mD.ft", "name"="millidarcy foot", "dimension"="L3", "is_si_unit"=TRUE, "category"="derived", "base_unit"="TD[API].m", "conversion_reference"="DERIVED", "is_exact"=TRUE, "a"=0.0, "b"=3.048e-16, "c"=1.01325, "d"=0.0, "underlying_def"="", "description"=""}, {"symbol"="mD.m", "name"="millidarcy metre", "dimension"="L3", "is_si_unit"=TRUE, "category"="derived", "base_unit"="TD[API].m", "conversion_reference"="DERIVED", "is_exact"=TRUE, "a"=0.0, "b"=1e-15, "c"=1.01325, "d"=0.0, "underlying_def"="", "description"=""}, {"symbol"="m3", "name"="cubic metre", "dimension"="L3", "is_si_unit"=TRUE, "category"="derived", "base_unit"="", "conversion_reference"="", "is_exact"=FALSE, "a"=0.0, "b"=0.0, "c"=0.0, "d"=0.0, "underlying_def"="", "description"=""}, {"symbol"="ft3", "name"="cubic foot", "dimension"="L3", "is_si_unit"=TRUE, "category"="derived", "base_unit"="m3", "conversion_reference"="DERIVED", "is_exact"=TRUE, "a"=0.0, "b"=0.028316846592, "c"=1.0, "d"=0.0, "underlying_def"="", "description"="The volume of a cube with sides of one foot (0.3048 m) in length"}, {"symbol"="in3", "name"="cubic inch", "dimension"="L3", "is_si_unit"=TRUE, "category"="derived", "base_unit"="m3", "conversion_reference"="DERIVED", "is_exact"=TRUE, "a"=0.0, "b"=1.6387064e-05, "c"=1.0, "d"=0.0, "underlying_def"="", "description"=""}, {"symbol"="mi3", "name"="cubic mile", "dimension"="L3", "is_si_unit"=TRUE, "category"="derived", "base_unit"="m3", "conversion_reference"="DERIVED", "is_exact"=TRUE, "a"=0.0, "b"=4168181825.4405794, "c"=1.0, "d"=0.0, "underlying_def"="", "description"=""}, {"symbol"="yd3", "name"="cubic yard", "dimension"="L3", "is_si_unit"=TRUE, "category"="derived", "base_unit"="m3", "conversion_reference"="DERIVED", "is_exact"=TRUE, "a"=0.0, "b"=0.764554857984, "c"=1.0, "d"=0.0, "underlying_def"="", "description"=""}, {"symbol"="hL", "name"="hectolitre", "dimension"="L3", "is_si_unit"=TRUE, "category"="prefixed", "base_unit"="m3", "conversion_reference"="DERIVED", "is_exact"=TRUE, "a"=0.0, "b"=0.1, "c"=1.0, "d"=0.0, "underlying_def"="", "description"=""}, {"symbol"="mL", "name"="millilitre", "dimension"="L3", "is_si_unit"=TRUE, "category"="prefixed", "base_unit"="m3", "conversion_reference"="DERIVED", "is_exact"=TRUE, "a"=0.0, "b"=1e-06, "c"=1.0, "d"=0.0, "underlying_def"="", "description"=""}, {"symbol"="m3/rad", "name"="cubic metre per radian", "dimension"="L3/A", "is_si_unit"=TRUE, "category"="derived", "base_unit"="", "conversion_reference"="", "is_exact"=FALSE, "a"=0.0, "b"=0.0, "c"=0.0, "d"=0.0, "underlying_def"="", "description"=""}, {"symbol"="ft3/rad", "name"="cubic foot per radian", "dimension"="L3/A", "is_si_unit"=TRUE, "category"="derived", "base_unit"="m3/rad", "conversion_reference"="DERIVED", "is_exact"=TRUE, "a"=0.0, "b"=0.028316846592, "c"=1.0, "d"=0.0, "underlying_def"="", "description"=""}, {"symbol"="m3/rev", "name"="cubic metre per revolution", "dimension"="L3/A", "is_si_unit"=TRUE, "category"="derived", "base_unit"="m3/rad", "conversion_reference"="DERIVED", "is_exact"=TRUE, "a"=0.0, "b"=1.0, "c"=2.0, "d"=0.0, "underlying_def"="", "description"=""}, {"symbol"="m3/kg", "name"="cubic metre per kilogram", "dimension"="L3/M", "is_si_unit"=TRUE, "category"="derived", "base_unit"="", "conversion_reference"="", "is_exact"=FALSE, "a"=0.0, "b"=0.0, "c"=0.0, "d"=0.0, "underlying_def"="", "description"=""}, {"symbol"="0.01 L/kg", "name"="litre per hundred kilogram", "dimension"="L3/M", "is_si_unit"=TRUE, "category"="derived", "base_unit"="m3/kg", "conversion_reference"="DERIVED", "is_exact"=TRUE, "a"=0.0, "b"=1e-05, "c"=1.0, "d"=0.0, "underlying_def"="", "description"=""}, {"symbol"="bbl/ton[UK]", "name"="barrel per UK ton-mass", "dimension"="L3/M", "is_si_unit"=TRUE, "category"="derived", "base_unit"="m3/kg", "conversion_reference"="DERIVED", "is_exact"=TRUE, "a"=0.0, "b"=0.158987294928, "c"=1016.0469088, "d"=0.0, "underlying_def"="", "description"=""}, {"symbol"="bbl/ton[US]", "name"="barrel per US ton-mass", "dimension"="L3/M", "is_si_unit"=TRUE, "category"="derived", "base_unit"="m3/kg", "conversion_reference"="DERIVED", "is_exact"=TRUE, "a"=0.0, "b"=0.158987294928, "c"=907.18474, "d"=0.0, "underlying_def"="", "description"=""}, {"symbol"="cm3/g", "name"="cubic centimetre per gram", "dimension"="L3/M", "is_si_unit"=TRUE, "category"="derived", "base_unit"="m3/kg", "conversion_reference"="DERIVED", "is_exact"=TRUE, "a"=0.0, "b"=0.001, "c"=1.0, "d"=0.0, "underlying_def"="", "description"=""}, {"symbol"="dm3/kg", "name"="cubic decimetre per kilogram", "dimension"="L3/M", "is_si_unit"=TRUE, "category"="derived", "base_unit"="m3/kg", "conversion_reference"="DERIVED", "is_exact"=TRUE, "a"=0.0, "b"=0.001, "c"=1.0, "d"=0.0, "underlying_def"="", "description"=""}, {"symbol"="dm3/t", "name"="cubic decimetre per ton", "dimension"="L3/M", "is_si_unit"=TRUE, "category"="derived", "base_unit"="m3/kg", "conversion_reference"="DERIVED", "is_exact"=TRUE, "a"=0.0, "b"=1e-06, "c"=1.0, "d"=0.0, "underlying_def"="", "description"=""}, {"symbol"="ft3/kg", "name"="cubic foot per kilogram", "dimension"="L3/M", "is_si_unit"=TRUE, "category"="derived", "base_unit"="m3/kg", "conversion_reference"="DERIVED", "is_exact"=TRUE, "a"=0.0, "b"=0.028316846592, "c"=1.0, "d"=0.0, "underlying_def"="", "description"=""}, {"symbol"="ft3/lbm", "name"="cubic foot per pound-mass", "dimension"="L3/M", "is_si_unit"=TRUE, "category"="derived", "base_unit"="m3/kg", "conversion_reference"="DERIVED", "is_exact"=TRUE, "a"=0.0, "b"=0.028316846592, "c"=0.45359237, "d"=0.0, "underlying_def"="", "description"=""}, {"symbol"="ft3/sack[94lbm]", "name"="cubic foot per 94-pound-sack", "dimension"="L3/M", "is_si_unit"=TRUE, "category"="derived", "base_unit"="m3/kg", "conversion_reference"="DERIVED", "is_exact"=TRUE, "a"=0.0, "b"=0.028316846592, "c"=42.63768278, "d"=0.0, "underlying_def"="", "description"=""}, {"symbol"="gal[UK]/lbm", "name"="UK gallon per pound-mass", "dimension"="L3/M", "is_si_unit"=TRUE, "category"="derived", "base_unit"="m3/kg", "conversion_reference"="DERIVED", "is_exact"=TRUE, "a"=0.0, "b"=0.00454609, "c"=0.45359237, "d"=0.0, 
